vi "Process.vi"(8 "error in":errorcluster, 11 "Instrument.Example":refnum<class "Instrument.Oxford1820.lvclass">) -> (0 "error out":errorcluster, 3 "Instrument.Example out":refnum<class "Instrument.Oxford1820.lvclass">)   [LabVIEW 2016, in "Instrument.Oxford1820.lvclass"]
doc: "---------------------------------------------------------------\nJKI State Machine Objects™\nhttp://jki.net/state-machine-objects/\nCopyright (C) 2005-2015, JKI <info@jki.net>\nALL RIGHTS RESERVED"
uses:
  Instrument.Oxford1820.lvclass
  C:/Program Files (x86)/National Instruments/LabVIEW 2016/vi.lib/JKI/JKI SMO/SMO/SMO.lvclass
  <vilib>/JKI/JKI SMO/SMO/Typedefs/Parent Call--Enum.ctl
  <instrlib>/Mercury iXX/Public/Libraries/Magnet/Controls/Switch Heater.ctl
  <userlib>/LevyLab/Levylab Instruments/Instrument Types/Cryostat/Instrument.Cryostat.lvclass
  <vilib>/JKI/JKI SMO/SMO/SMO.lvclass
  <instrlib>/Mercury iXX/Public/Libraries/Magnet.lvlib
panel:
  # "For instructions on how to use the JKI State Machine Objects, examples and video tutorials, visit:\nhttp://jki.net/state-machine-objects/\n\nJKI State Machine Objects™\nhttp://jki.net/state-machine-objects/\nCopyright (C) 2005-2015, JKI <info@jki.net>\nALL RIGHTS RESERVED"
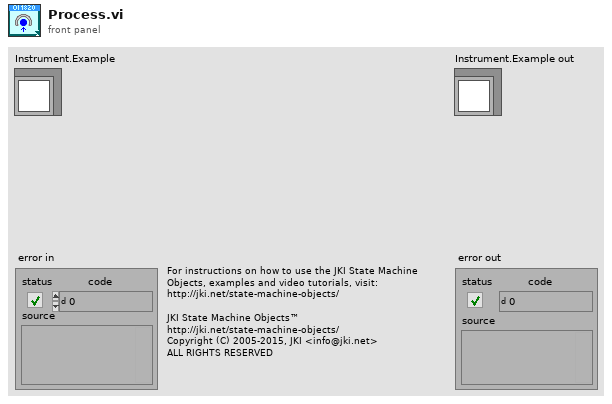
[diagram p1: front panel]
types:
  T1 = typedef "SMO.lvclass/Parent Call--Enum.ctl" = enum16{"Allows parent to run", "Does not request parent to run"}
  T2 = enum32{"invalid app kind", "Development System", "Run Time System", "Student Edition", "Embedded LabVIEW", "Evaluation", "Custom"}
  T3 = enum32{"Invalid", "Standard", "Closed", "Hidden", "Minimized", "Maximized"}
  T4 = enum32{"Bad", "Idle", "Run top level", "Running"}
  T5 = typedef "Mercury iXX.lvlib/Magnet.lvlib/Switch Heater.ctl" = string
  T6 = cluster{"Core":cluster{"Current VI Reference":refnum<vi>, "Close Panel on Exit?":bool, "error":errorcluster}, "Self Reference":refnum<class "Instrument.Oxford1820.lvclass">, "Field (T)":dbl, "Field Rate (T/min)":dbl, "persistent":bool, "Running Step":i32, "sequence":string[]}
  T7 = cluster{"Current VI Reference":refnum<vi>, "Close Panel on Exit?":bool, "error":errorcluster}
  T8 = typedef "SMO.lvclass/Protected Events.ctl" = cluster{"StopProcesses":refnum<user-event>, "AbortProcesses":refnum<user-event>, "Config Changed":refnum<user-event>, "Dependency":refnum<user-event>}
  T9 = typedef "Instrument.Oxford1820.lvclass/PrivateEvents--Cluster.ctl" = cluster{"SequenceSetMagnetField":refnum<user-event>}
  T10 = cluster{"Holding":bool, "Ramp to Setpoint":bool, "Ramp to Zero":bool, "Clamp":bool}
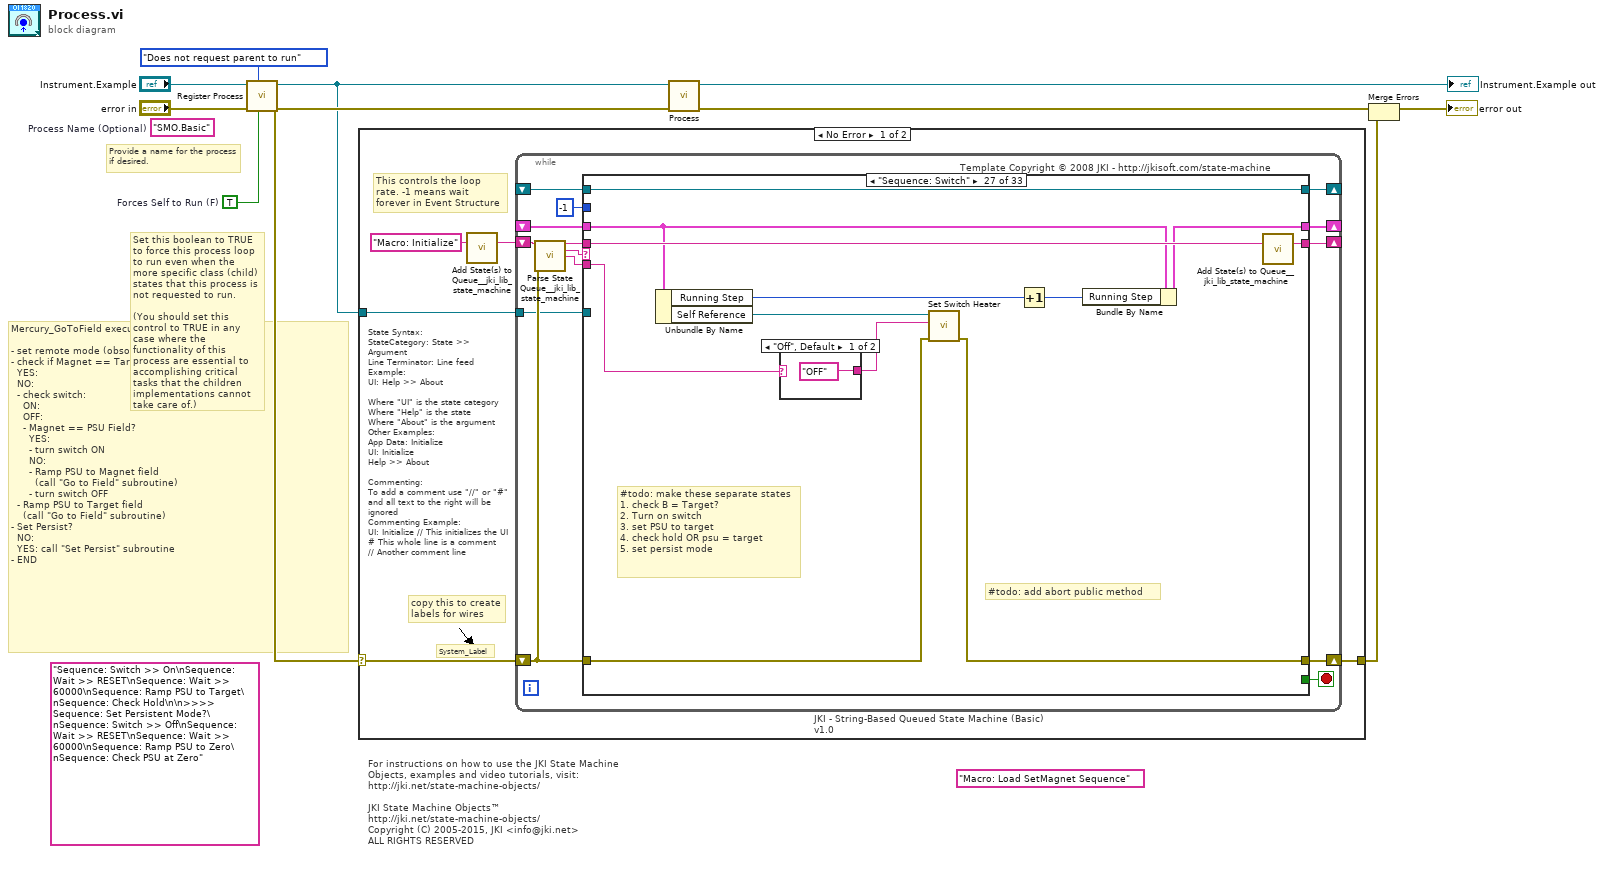
[diagram p0: block diagram]
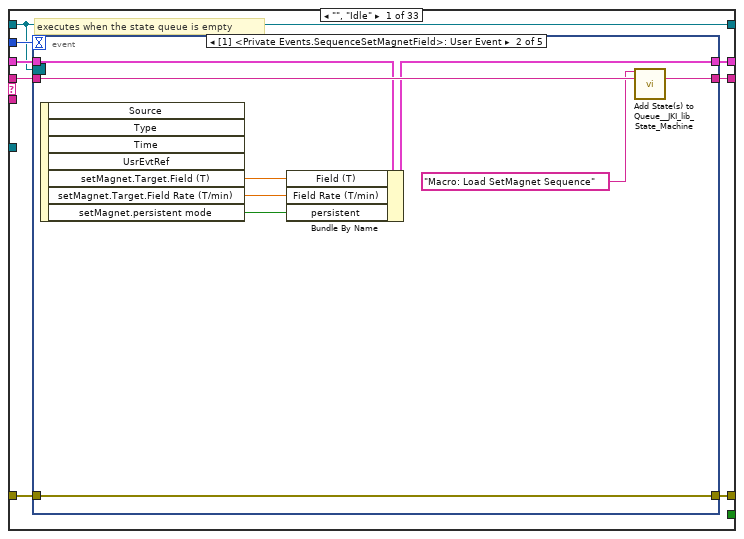
[diagram p2: hidden frame]
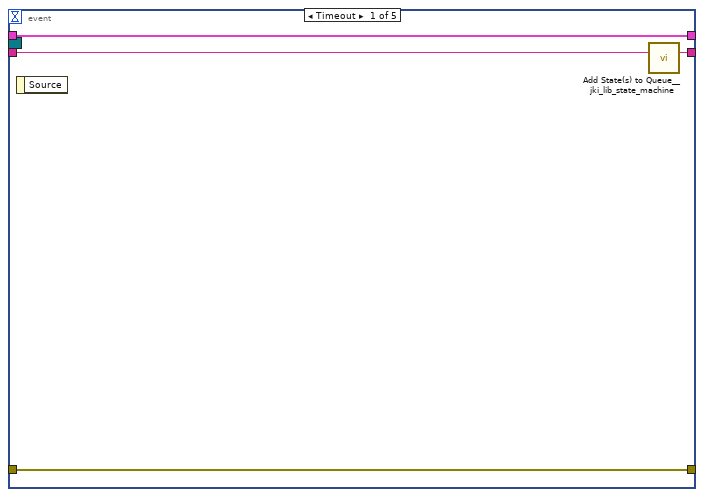
[diagram p3: hidden frame]
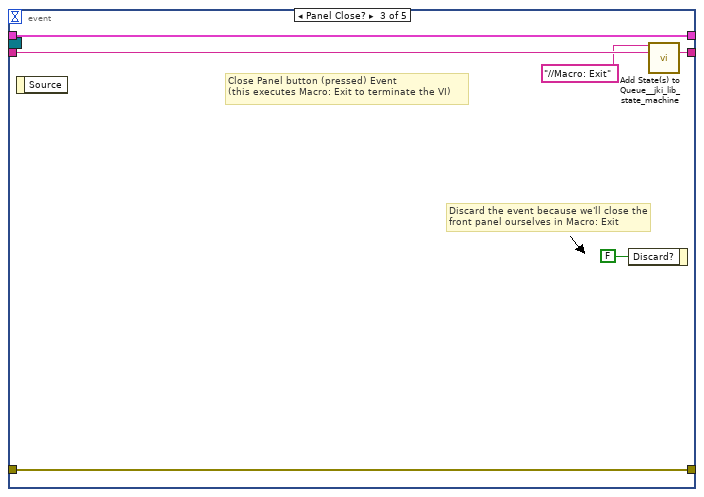
[diagram p4: hidden frame]
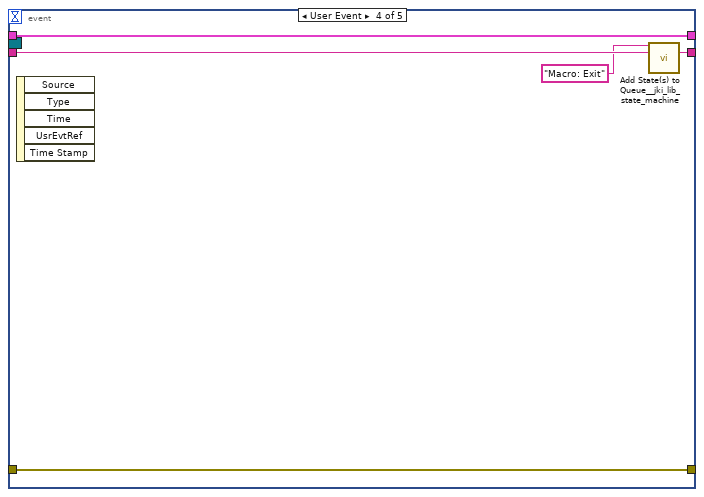
[diagram p5: hidden frame]
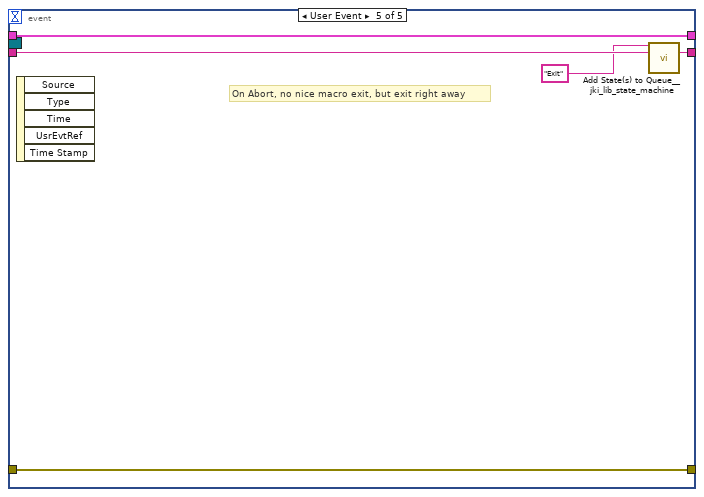
[diagram p6: hidden frame]
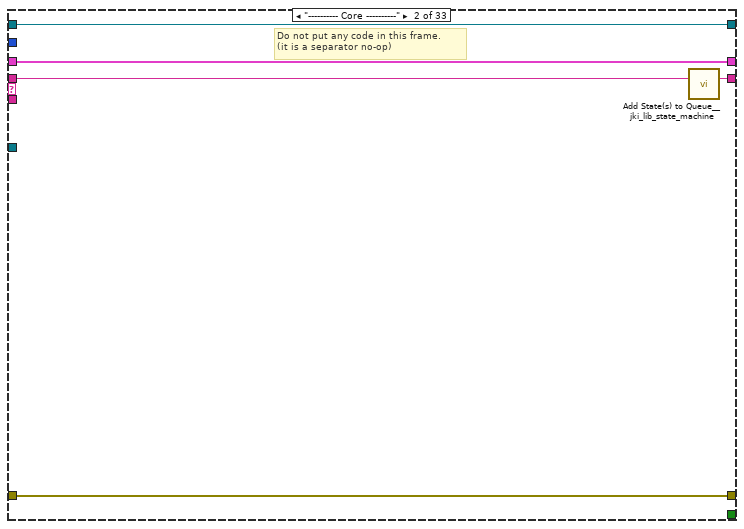
[diagram p7: hidden frame]
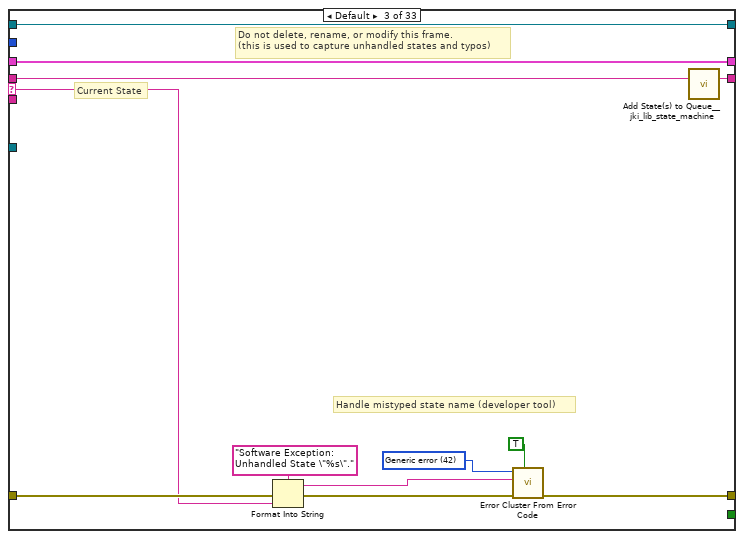
[diagram p8: hidden frame]
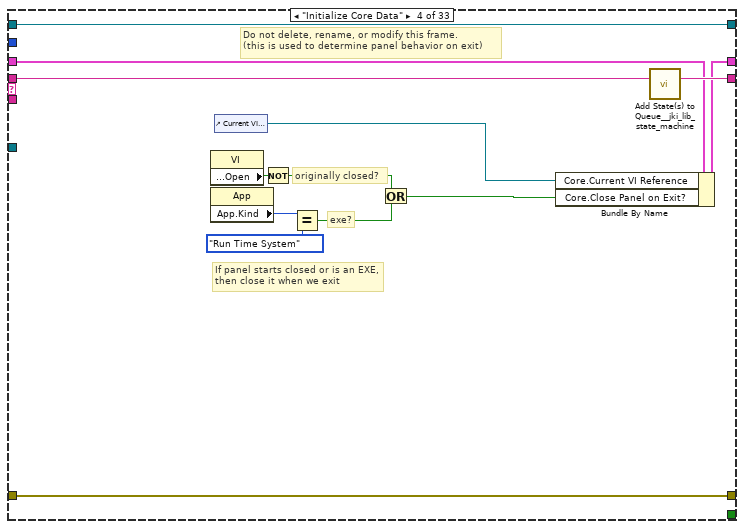
[diagram p9: hidden frame]
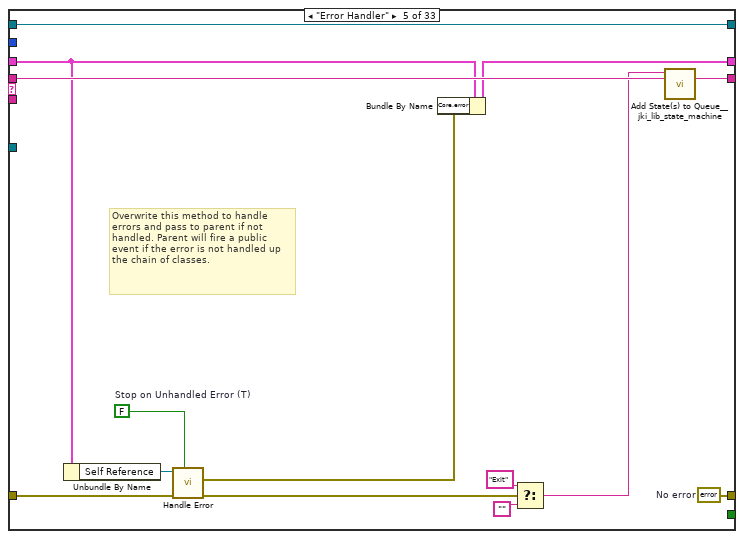
[diagram p10: hidden frame]
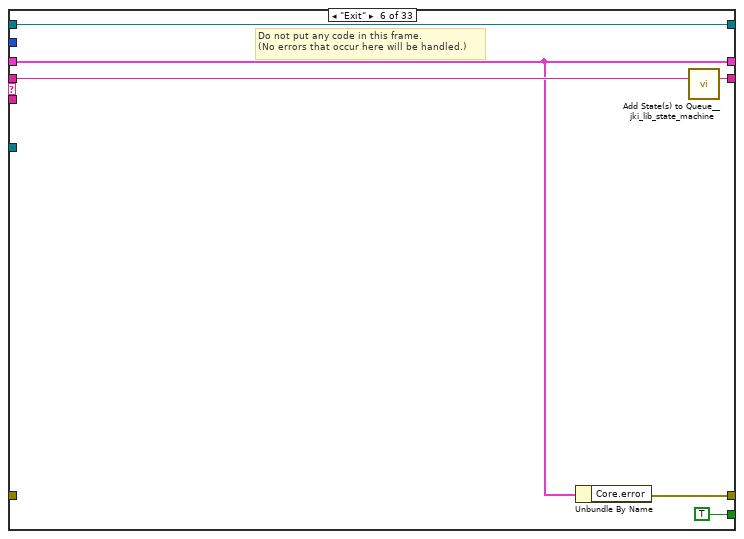
[diagram p11: hidden frame]
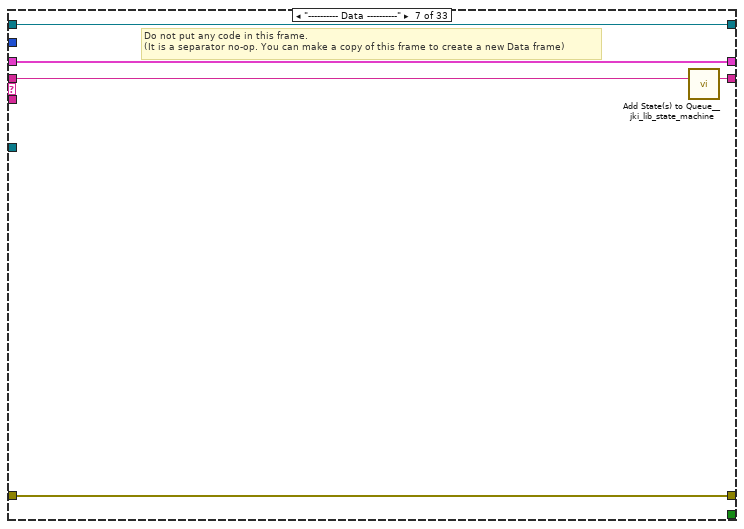
[diagram p12: hidden frame]
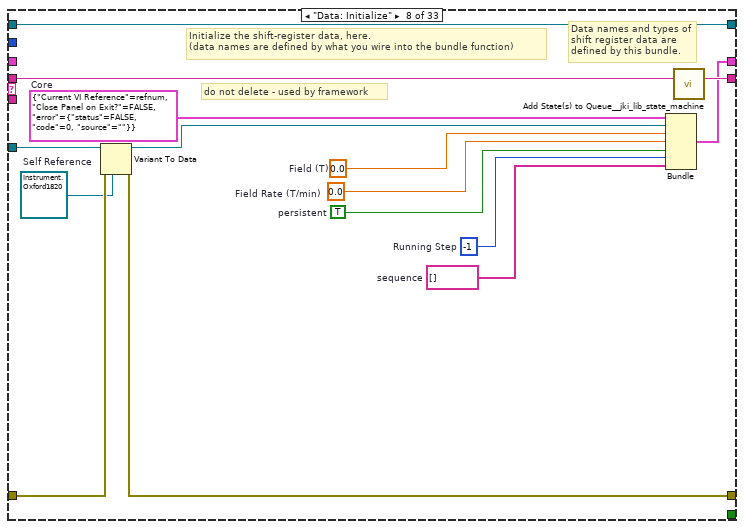
[diagram p13: hidden frame]
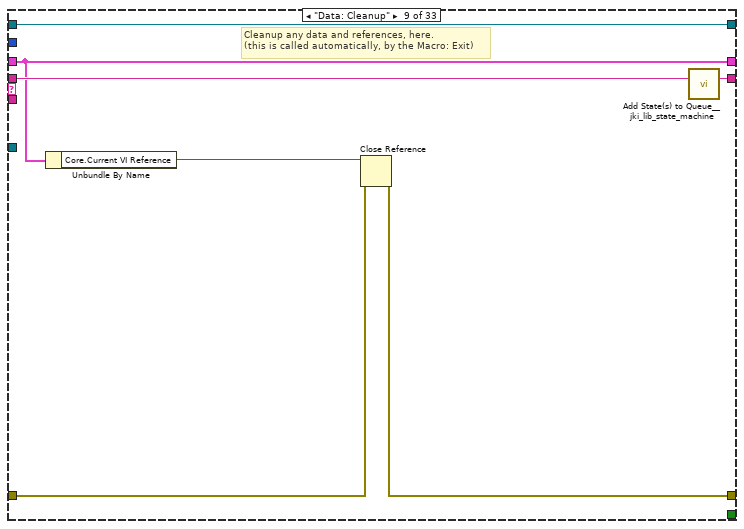
[diagram p14: hidden frame]
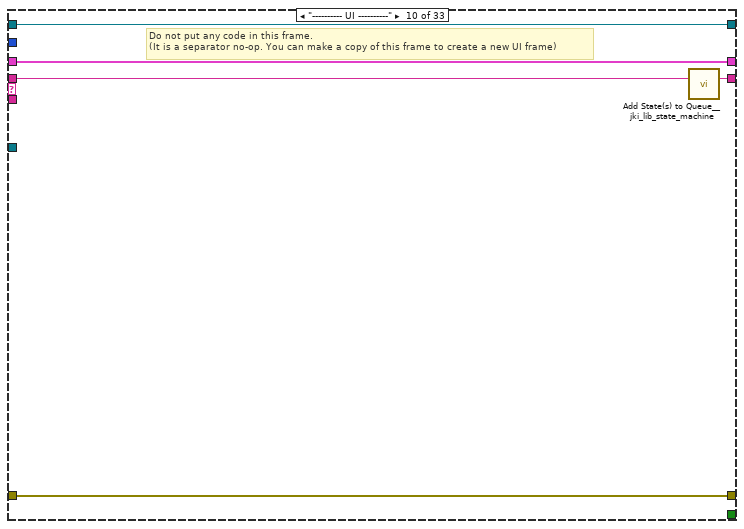
[diagram p15: hidden frame]
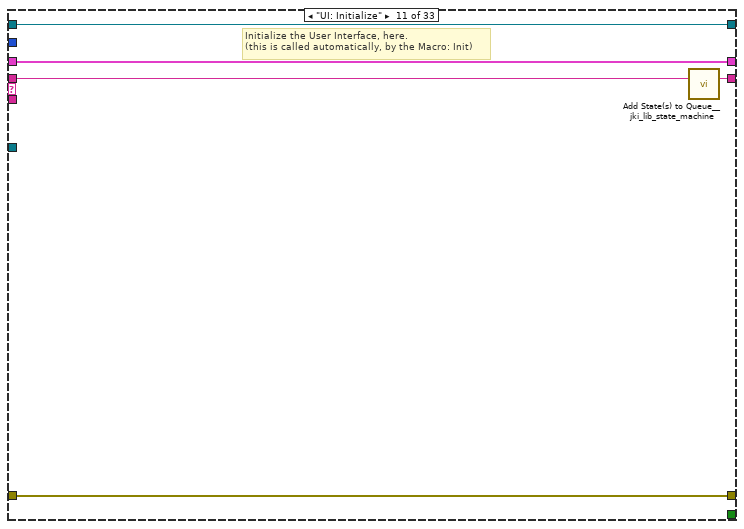
[diagram p16: hidden frame]
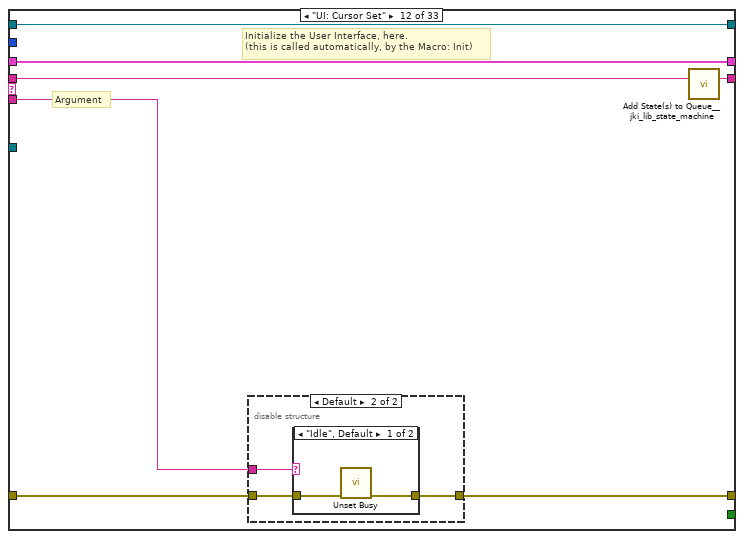
[diagram p17: hidden frame]
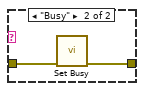
[diagram p19: hidden frame]
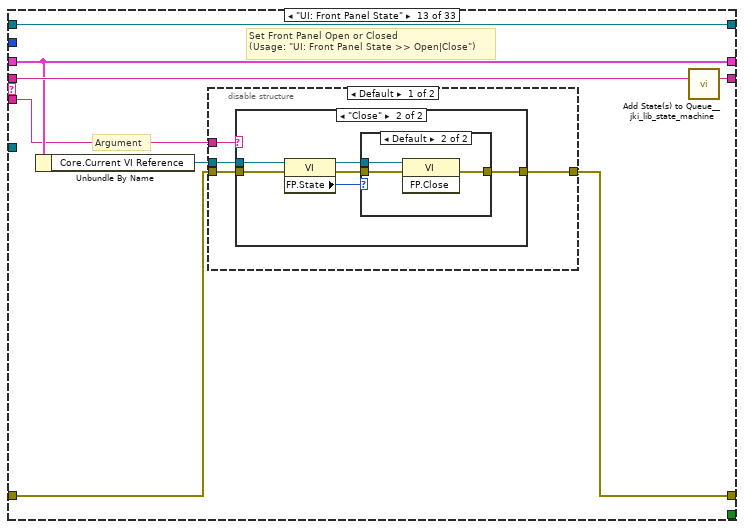
[diagram p20: hidden frame]
diagram:
  (unwired) "Macro: Load SetMagnet Sequence" ("State(s) at Back (\"\")")
  (unwired) "Sequence: Switch >> On\nSequence: Wait >> RESET\nSequence: Wait >> 60000\nSequence: Ramp PSU to Target\nSequence: Check Hold\n\n>>>> Sequence: Set Persistent Mode?\nSequence: Switch >> Off\nSequence: Wait >> RESET\nSequence: Wait >> 60000\nSequence: Ramp PSU to Zero\nSequence: Check PSU at Zero" ("State(s) in Front (\"\")")
  w1 = TRUE  # Forces Self to Run (F)
  (unwired) "SMO.Basic"  # Process Name (Optional)
  # "Mercury_GoToField executes the following states:\n\n- set remote mode (obsolete?)\n- check if Magnet == Target.\n  YES:\n  NO:\n  - check switch:\n    ON:\n    OFF:\n    - Magnet == PSU Field?\n      YES:\n      - turn switch ON\n      NO:\n      - Ramp PSU to Magnet field\n        (call \"Go to Field\" subroutine)\n      - turn switch OFF\n  - Ramp PSU to Target field\n    (call \"Go to Field\" subroutine)\n- Set Persist?\n  NO:\n  YES: call \"Set Persist\" subroutine\n- END"
  # "Provide a name for the process\nif desired."
  # "Set this boolean to TRUE to force this process loop to run even when the more specific class (child) states that this process is not requested to run.\n\n(You should set this control to TRUE in any case where the functionality of this process are essential to accomplishing critical tasks that the children implementations cannot take care of.)"
  # "For instructions on how to use the JKI State Machine Objects, examples and video tutorials, visit:\nhttp://jki.net/state-machine-objects/\n\nJKI State Machine Objects™\nhttp://jki.net/state-machine-objects/\nCopyright (C) 2005-2015, JKI <info@jki.net>\nALL RIGHTS RESERVED"
  n1 = call <vilib>:"Register Process.vi"("Forces Self to Run (F)"=w1, "Parent Call"=Parent_Call--Enum."Does not request parent to run", "error in (no error)"="error in", "SMO"="Instrument.Example") -> ("error out"=w7:errorcluster, "SMO out"=w6:refnum<class "Instrument.Oxford1820.lvclass">)  [unwired: 6 in]
  n2 = case shown="No Error" w7 {
    selector: w7 -> [w12 w472]
    tunnel: w6 -> [w13 _]
    tunnel: [w11 w472] -> w3
    frame No Error {
      # "State Syntax:\nStateCategory: State >> Argument\nLine Terminator: Line feed\nExample:\nUI: Help >> About\n\nWhere \"UI\" is the state category\nWhere \"Help\" is the state\nWhere \"About\" is the argument\nOther Examples:\nApp Data: Initialize\nUI: Initialize\nHelp >> About\n\nCommenting:\nTo add a comment use \"//\" or \"#\" and all text to the right will be ignored\nCommenting Example:\nUI: Initialize // This initializes the UI\n# This whole line is a comment\n// Another comment line"
      # "copy this to create labels for wires"
      # "This controls the loop rate. -1 means wait forever in Event Structure"
      # "System_Label"
      n3 = call <vilib>:"Add State(s) to Queue__jki_lib_state_machine.vi"("State(s) in (\"\")"="Macro: Initialize") -> ("States Out"=w15:string)  [unwired: 14 in]
      n4 = while "JKI - String-Based Queued State Machine (Basic) v1.0" {
        shift-right: [w22] -> _
        shift-left: _ -> [w21]
        shift-right: [w25] -> w11
        shift-left: w12 -> [w19]
        shift-right: [w24] -> _
        shift-left: w15 -> [w26]
        tunnel: w13 -> [w18]
        shift-right: [w17] -> _
        shift-left: _ -> [w16]
        stop <- w23 stop-if-true
        # "Template Copyright © 2008 JKI - http://jkisoft.com/state-machine"
        n5 = call <vilib>:"Parse State Queue__jki_lib_state_machine.vi"("State Queue"=w26, "Error In (no error)"=w19) -> ("Remaining States"=w28:string, "Current State"=w29:string, "Arguments"=w27:string)  [unwired: 11 in]
        n6 = case shown="\"Sequence: Switch\"" w29 {
          selector: w29 -> [_ _ w73 _ _ _ _ _ _ _ _ _ _ _ _ _ _ _ _ _ _ _ _ _ _ _ _ _ _ _ _ _ _]
          tunnel: w28 -> [w37 w71 w77 w96 w110 w116 w121 w136 w143 w148 w153 w160 w176 w208 w222 w236 w253 w268 w273 w284 w289 w302 w308 w317 w324 w338 w370 w388 w412 w432 w445 w459 w467]
          tunnel: w27 -> [_ _ _ _ _ _ _ _ _ _ _ w154 w170 _ _ _ _ _ _ _ _ _ _ _ _ _ w361 w373 _ _ _ _ _]
          tunnel: w21 -> [w35 w68 w75 w87 w104 w112 w118 _ w138 w145 w151 w158 w172 w205 w218 w227 w238 w264 w270 w281 w286 w300 w306 w311 w320 w335 w363 w385 w404 w429 w435 w456 w464]
          tunnel: [w34 w69 w79 w93 w105 w111 w119 w132 w139 w146 w150 w155 w173 w206 w220 w234 w251 w266 w271 w275 w287 w295 w304 w314 w321 w325 w359 w376 w400 w423 w440 w450 w461] -> w25
          tunnel: w19 -> [w33 w69 w78 w93 w106 _ w119 w133 w140 w146 w150 w156 w174 w206 w220 w234 w251 w266 w271 w276 w287 w296 w304 w314 w321 w326 w367 w375 w406 w424 w441 w451 w462]
          tunnel: [w36 w70 w76 w95 w109 w115 w120 w135 w142 w147 w152 w159 w175 w207 w221 w235 w252 w267 w272 w283 w288 w301 w307 w316 w323 w337 w369 w387 w411 w431 w444 w458 w466] -> w24
          tunnel: [_ _ _ _ _ TRUE _ _ _ _ _ _ _ _ _ _ _ _ _ _ _ _ _ _ _ _ _ _ _ _ _ _ _] -> w23
          tunnel: [w32 w68 w75 w94 w103 w112 w118 w134 w138 w145 w151 w158 w172 w205 w218 w227 w249 w262 w270 w281 w286 w300 w306 w310 w319 w335 w362 w384 w403 w428 w433 w455 w464] -> w22
          tunnel: -1 ("Timeout") -> [w31 _ _ _ _ _ _ _ _ _ _ _ _ _ _ _ _ _ _ _ _ _ _ _ _ _ _ _ _ _ _ _ _]
          tunnel: w18 -> [_ _ _ _ _ _ _ w130 _ _ _ _ _ _ _ _ _ _ _ _ _ _ _ _ _ _ _ _ _ _ _ _ _]
          tunnel: [w30 w67 w72 w84 w108 w113 w117 w128 w137 w144 w149 w157 w169 w204 w219 w228 w250 w265 w269 w282 w285 w299 w305 w315 w322 w336 w368 w386 w410 w430 w443 w457 w465] -> w17
          tunnel: w16 -> [w30 w67 w72 w84 w108 w113 w117 w128 w137 w144 w149 w157 w169 w204 w219 w228 w250 w265 w269 w282 w285 _ w305 w315 w322 w336 w368 w386 w410 w430 w443 w457 w465]
          frame "", "Idle" {
            # "executes when the state queue is empty"
            n7 = event shown="[1] <Private Events.SequenceSetMagnetField>: User Event" {
              selector: w30 -> [_ _ _ _ _]
              dyn-events: _ -> [_ _ _ _ _]
              timeout: w31 -> [_ _ _ _ _]
              tunnel: w37 -> [w41 w48 w56 w61 w66]
              tunnel: [w40 w49 w55 w60 w65] -> w36
              tunnel: w35 -> [w38 w44 w53 w58 w63]
              tunnel: [w39 w50 w54 w59 w64] -> w34
              tunnel: w33 -> [w39 w50 w54 w59 w64]
              tunnel: [w38 w43 w53 w58 w63] -> w32
              event Timeout {
                n8 = event-data() -> ()  [unwired: 1 in, 1 out]
                n9 = call <vilib>:"Add State(s) to Queue__jki_lib_state_machine.vi"("State(s) in (\"\")"=w41) -> ("States Out"=w40:string)  [unwired: 14 in]
              }
              event User Event {
                n10 = event-data() -> ("setMagnet.Target.Field (T)"=w47:dbl, "setMagnet.Target.Field Rate (T/min)"=w46:dbl, "setMagnet.persistent mode"=w45:bool)  [unwired: 1 in, 4 out]
                n11 = Bundle By Name(cluster=w44, "Field (T)"=w47, "Field Rate (T/min)"=w46, "persistent"=w45) -> (w43:T6)
                n12 = call <vilib>:"Add State(s) to Queue__JKI_lib_State_Machine.vi"("State(s) in Front (\"\")"="Macro: Load SetMagnet Sequence" ("State(s) at Back (\"\")"), "State(s) in (\"\")"=w48) -> ("States Out"=w49:string)  [unwired: 13 in]
              }
              event Panel Close? {
                # "Discard the event because we'll close the front panel ourselves in Macro: Exit"
                # "Close Panel button (pressed) Event\n(this executes Macro: Exit to terminate the VI)"
                n13 = event-data() -> ()  [unwired: 1 in, 1 out]
                n14 = event-data("Discard?"=FALSE) -> ()  [unwired: 1 in, 1 out]
                n15 = call <vilib>:"Add State(s) to Queue__jki_lib_state_machine.vi"("State(s) in Front (\"\")"="//Macro: Exit", "State(s) in (\"\")"=w56) -> ("States Out"=w55:string)  [unwired: 13 in]
              }
              event User Event {
                n16 = event-data() -> ()  [unwired: 1 in, 5 out]
                n17 = call <vilib>:"Add State(s) to Queue__jki_lib_state_machine.vi"("State(s) in Front (\"\")"="Macro: Exit", "State(s) in (\"\")"=w61) -> ("States Out"=w60:string)  [unwired: 13 in]
              }
              event User Event {
                # "On Abort, no nice macro exit, but exit right away"
                n18 = event-data() -> ()  [unwired: 1 in, 5 out]
                n19 = call <vilib>:"Add State(s) to Queue__jki_lib_state_machine.vi"("State(s) in Front (\"\")"="Exit", "State(s) in (\"\")"=w66) -> ("States Out"=w65:string)  [unwired: 13 in]
              }
            }
          }
          frame "---------- Core ----------" {
            # "Do not put any code in this frame.\n(it is a separator no-op)"
            n20 = call <vilib>:"Add State(s) to Queue__jki_lib_state_machine.vi"("State(s) in (\"\")"=w71) -> ("States Out"=w70:string)  [unwired: 14 in]
          }
          frame Default {
            w82 = 42 items=["No error", "Argument error", "Memory is full", "Out of zone", "End of file", "File already open", "Generic file I/O error", "File not found", "File permission error", "Disk is full", "Duplicate path", "Too many files open", "System feature not enabled", "Resource file not found", "Cannot add resource", "Resource not found", "Image not found", "Image memory error", "Pen does not exist", "Config type invalid", "Config token not found", "Config parse error", "Config memory error", "Bad external code format", "Bad external code offset", "External code not present", "Null window", "Destroy window error", "Null menu", "Print aborted", "Bad print record", "Print driver error", "Windows error during printing", "Memory error during printing", "Print dialog error", "Generic print error", "Invalid device refnum", "Device not found", "Device parameter error", "Device unit error", "Cannot open device", "Device call aborted", "Generic error", "Cancelled by user", "Object ID too low", "Object ID too high", "Object not in heap", "Unknown heap", "Unknown object (invalid DefProc)", "Unknown object (DefProc not in table)", "Message out of range", "Invalid (null) method", "Unknown message", "Manager call not supported", "Bad address", "Network operation in progress", "Network operation timed out", "Connection is busy", "Network attribute not supported", "Network error", "Address in use", "System out of memory", "Connection aborted", "Connection refused", "Not connected", "Already connected", "Connection closed", "Initialization error (interapplication manager)", "Bad occurrence", "Wait on unbound occurrence handler", "Occurrence queue overflow", "Datalog type conflict", "Unused", "Unrecognized type (interapplication manager)", "Memory corrupt", "Failed to make temporary DLL", "Old CIN version", "Drag socket not found", "Failed to load drop-object", "Failed to register OLE object", "Failed to release OLE object", "Format specifier type mismatch", "Unknown format specifier", "Too few format specifiers", "Too many format specifiers", "Scan failed", "Newer CIN version", "Error converting to variant", "Runtime menu error", "Password tampered", "Variant attribute not found", "Incompatible variant data type", "Event data is not available", "Event Store is not present", "Occurrence is not found", "Event Queue is not created", "Event info is not available", "Refnum passed is NULL", "Error retrieving Class GUID", "Error retrieving CoClass GUID", "Error retrieving TypeLib GUID.", "Bad built application magic bytes.", "Specific driver is different from the specific driver associated with the Logical Name.", "There is no session opened to the class driver.", "Max Error", "MAX - Error with config objects", "MAX - Error loading configuration", "MAX - Group not supported"]
            # "Current State"
            # "Do not delete, rename, or modify this frame.\n(this is used to capture unhandled states and typos)"
            # "Handle mistyped state name (developer tool)"
            n21 = Format Into String(format string="Software Exception: Unhandled State \"%s\"." ("message"), error in=w78, w73) -> (resulting string=w81:string, error out=w80:errorcluster)  [unwired: 1 in]
            n22 = call <vilib>:"Error Cluster From Error Code.vi"("show call chain? (False)"=TRUE, "error in (no error)"=w80, "error message (\"\")"=w81, "error code (0)"=w82) -> ("error out"=w79:errorcluster)  [unwired: 5 in]
            n23 = call <vilib>:"Add State(s) to Queue__jki_lib_state_machine.vi"("State(s) in (\"\")"=w77) -> ("States Out"=w76:string)  [unwired: 14 in]
          }
          frame "Initialize Core Data" {
            # "Do not delete, rename, or modify this frame.\n(this is used to determine panel behavior on exit)"
            # "originally closed?"
            # "exe?"
            # "If panel starts closed or is an EXE, then close it when we exit"
            n24 = property class="VI"() -> ("Front Panel.Open"=w92:bool)  [unwired: 2 in, 2 out]
            n25 = property class="App"() -> ("App.Kind"=w91:T2)  [unwired: 2 in, 2 out]
            n26 = control-ref of="Current VI Reference"() -> (w85:refnum<vi>)
            n27 = Not(x=w92) -> (.not. x?=w89:bool)
            n28 = Equal?(x=w91, y=T2."Run Time System" ("Application:Kind")) -> (x = y?=w88:bool)
            n29 = Or(x=w89, y=w88) -> (x .or. y?=w86:bool)
            n30 = Bundle By Name(cluster=w87, "Core.Current VI Reference"=w85, "Core.Close Panel on Exit?"=w86) -> (w94:T6)
            n31 = call <vilib>:"Add State(s) to Queue__jki_lib_state_machine.vi"("State(s) in (\"\")"=w96) -> ("States Out"=w95:string)  [unwired: 14 in]
          }
          frame "Error Handler" {
            w97 = FALSE  # Stop on Unhandled Error (T)
            w105 = errorcluster {"status"=FALSE, "code"=0, "source"=""}  # No error
            # "Overwrite this method to handle errors and pass to parent if not handled. Parent will fire a public event if the error is not handled up the chain of classes."
            n32 = Unbundle By Name(w104) -> ("Self Reference"=w107:refnum<class "Instrument.Oxford1820.lvclass">)
            n33 = call-dynamic "Handle Error.vi"("Stop on Unhandled Error (T)"=w97, "error in"=w106, "LevyLab"=w107) -> ("handling error"=w98:errorcluster, "Unhandled error"=w101:errorcluster)  [unwired: 6 in, 1 out]
            n34 = Bundle By Name(cluster=w104, "Core.error"=w101) -> (w103:T6)
            n35 = Select(t="Exit", s=w98, f="") -> (s? t:f=w102:string)
            n36 = call <vilib>:"Add State(s) to Queue__jki_lib_state_machine.vi"("State(s) in Front (\"\")"=w102, "State(s) in (\"\")"=w110) -> ("States Out"=w109:string)  [unwired: 13 in]
          }
          frame "Exit" {
            # "Do not put any code in this frame.\n(No errors that occur here will be handled.)"
            n37 = Unbundle By Name(w112) -> ("Core.error"=w111:errorcluster)
            n38 = call <vilib>:"Add State(s) to Queue__jki_lib_state_machine.vi"("State(s) in (\"\")"=w116) -> ("States Out"=w115:string)  [unwired: 14 in]
          }
          frame "---------- Data ----------" {
            # "Do not put any code in this frame.\n(It is a separator no-op. You can make a copy of this frame to create a new Data frame)"
            n39 = call <vilib>:"Add State(s) to Queue__jki_lib_state_machine.vi"("State(s) in (\"\")"=w121) -> ("States Out"=w120:string)  [unwired: 14 in]
          }
          frame "Data: Initialize" {
            w122 = string[] []  # sequence
            w123 = -1  # Running Step
            w124 = TRUE  # persistent
            w125 = 0.0  # Field Rate (T/min)
            w126 = 0.0  # Field (T)
            w127 = T7 {"Current VI Reference"=refnum, "Close Panel on Exit?"=FALSE, "error"={"status"=FALSE, "code"=0, "source"=""}}  # Core
            w131 = refnum<class "Instrument.Oxford1820.lvclass"> refnum  # Self Reference
            # "do not delete - used by framework"
            # "Data names and types of shift register data are defined by this bundle."
            # "Initialize the shift-register data, here.\n(data names are defined by what you wire into the bundle function)"
            n40 = Variant To Data(error in=w133, type=w131, Variant=w130) -> (data=w129:refnum<class "Instrument.Oxford1820.lvclass">, error out=w132:errorcluster)
            n41 = Bundle("Core"=w127, "Self Reference"=w129, "Field (T)"=w126, "Field Rate (T/min)"=w125, "persistent"=w124, "Running Step"=w123, "sequence"=w122) -> (w134:T6)  [unwired: 1 in]
            n42 = call <vilib>:"Add State(s) to Queue__jki_lib_state_machine.vi"("State(s) in (\"\")"=w136) -> ("States Out"=w135:string)  [unwired: 14 in]
          }
          frame "Data: Cleanup" {
            # "Cleanup any data and references, here.\n(this is called automatically, by the Macro: Exit)"
            n43 = Unbundle By Name(w138) -> ("Core.Current VI Reference"=w141:refnum<vi>)
            n44 = Close Reference(reference=w141, error in (no error)=w140) -> (error out=w139:errorcluster)
            n45 = call <vilib>:"Add State(s) to Queue__jki_lib_state_machine.vi"("State(s) in (\"\")"=w143) -> ("States Out"=w142:string)  [unwired: 14 in]
          }
          frame "---------- UI ----------" {
            # "Do not put any code in this frame.\n(It is a separator no-op. You can make a copy of this frame to create a new UI frame)"
            n46 = call <vilib>:"Add State(s) to Queue__jki_lib_state_machine.vi"("State(s) in (\"\")"=w148) -> ("States Out"=w147:string)  [unwired: 14 in]
          }
          frame "UI: Initialize" {
            # "Initialize the User Interface, here.\n(this is called automatically, by the Macro: Init)"
            n47 = call <vilib>:"Add State(s) to Queue__jki_lib_state_machine.vi"("State(s) in (\"\")"=w153) -> ("States Out"=w152:string)  [unwired: 14 in]
          }
          frame "UI: Cursor Set" {
            # "Argument"
            # "Initialize the User Interface, here.\n(this is called automatically, by the Macro: Init)"
            n48 = disable-structure shown="Default" {
              disable-tunnel: w156 -> [w161 w164]
              disable-tunnel: [w161 w163] -> w155
              disable-tunnel: w154 -> [_ w162]
              frame condition #0 {
              }
              frame condition #1 (active) {
                n49 = case shown="\"Idle\", Default" w162 {
                  tunnel: w164 -> [w166 w168]
                  tunnel: [w165 w167] -> w163
                  frame "Idle", Default {
                    n50 = call <vilib>:"Unset Busy.vi"("error in (no error)"=w166) -> ("error out"=w165:errorcluster)  [unwired: 10 in]
                  }
                  frame "Busy" {
                    n51 = call <vilib>:"Set Busy.vi"("error in (no error)"=w168) -> ("error out"=w167:errorcluster)  [unwired: 9 in, 1 out]
                  }
                }
              }
            }
            n52 = call <vilib>:"Add State(s) to Queue__jki_lib_state_machine.vi"("State(s) in (\"\")"=w160) -> ("States Out"=w159:string)  [unwired: 14 in]
          }
          frame "UI: Front Panel State" {
            # "Argument"
            # "Set Front Panel Open or Closed\n(Usage: \"UI: Front Panel State >> Open|Close\")"
            n53 = Unbundle By Name(w172) -> ("Core.Current VI Reference"=w171:refnum<vi>)
            n54 = disable-structure shown="Default" {
              disable-tunnel: w174 -> [w180 w203]
              disable-tunnel: [w179 w203] -> w173
              disable-tunnel: w171 -> [w178 _]
              disable-tunnel: w170 -> [w177 _]
              frame condition #0 (active) {
                n55 = case shown="\"Close\"" w177 {
                  tunnel: w180 -> [w184 w197]
                  tunnel: [w186 w198] -> w179
                  tunnel: w178 -> [w185 w195]
                  frame "Open", Default {
                    n56 = property class="VI"(reference=w185, error in=w184) -> (reference out=w182:refnum<vi>, error out=w183:errorcluster, "FP.State"=w181:T3)
                    n57 = case shown="\"Closed\"" w181 {
                      tunnel: [w189 w192] -> w186
                      tunnel: w183 -> [w188 w192]
                      tunnel: w182 -> [w187 _]
                      frame "Closed" {
                        n58 = invoke class="VI" method="FP.Open"(reference=w187, error in=w188, "Activate"=TRUE, "State"=T3."Standard") -> (error out=w189:errorcluster)  [unwired: 1 in, 4 out]
                      }
                      frame Default {
                      }
                    }
                  }
                  frame "Close" {
                    n59 = property class="VI"(reference=w195, error in=w197) -> (reference out=w194:refnum<vi>, error out=w196:errorcluster, "FP.State"=w193:T3)
                    n60 = case shown="Default" w193 {
                      tunnel: [w199 w202] -> w198
                      tunnel: w196 -> [w199 w201]
                      tunnel: w194 -> [_ w200]
                      frame "Invalid", "Closed" {
                      }
                      frame Default {
                        n61 = invoke class="VI" method="FP.Close"(reference=w200, error in=w201) -> (error out=w202:errorcluster)  [unwired: 1 in, 2 out]
                      }
                    }
                  }
                }
              }
              frame condition #1 {
              }
            }
            n62 = call <vilib>:"Add State(s) to Queue__jki_lib_state_machine.vi"("State(s) in (\"\")"=w176) -> ("States Out"=w175:string)  [unwired: 14 in]
          }
          frame "---------- Macro ----------" {
            # "Do not put any code in this frame.\n(It is a separator no-op. You can make a copy of this frame to create a new Macro frame)"
            n63 = call <vilib>:"Add State(s) to Queue__jki_lib_state_machine.vi"("State(s) in (\"\")"=w208) -> ("States Out"=w207:string)  [unwired: 14 in]
          }
          frame "Macro: Initialize" {
            w213 = "//UI: Initialize\n//UI: Front Panel State >> Open"  # //UI: Initialize //UI: Front Panel State >> Open
            w209 = "Process: Sync"
            # "Initialization Macro\n(This is called once, when the VI starts)"
            n64 = control-ref of="This VI"() -> (w211:refnum<vi>)
            n65 = property class="VI"(reference=w211) -> ("Exec.State"=w210:T4)  [unwired: 1 in, 2 out]
            n66 = Equal?(x=w210, y=T4."Run top level") -> (x = y?=w216:bool)
            n67 = Select(t=w209, s=w216, f="") -> ()  [unwired: 1 out]
            n68 = call <vilib>:"Add State(s) to Queue__jki_lib_state_machine.vi"("State(s) in Front (\"\")"="Data: Initialize\nInitialize Core Data\nEvents: Register", "State(s) in (\"\")"=w209, "State(s) at Back (\"\")"=w213) -> ("States Out"=w212:string)  [unwired: 12 in]
            n69 = call <vilib>:"Add State(s) to Queue__jki_lib_state_machine.vi"("State(s) in Front (\"\")"=w212, "State(s) in (\"\")"=w222) -> ("States Out"=w221:string)  [unwired: 13 in]
          }
          frame "Macro: Exit" {
            # "Exit Macro\n(This is called once, when the VI exits)"
            n70 = Unbundle By Name(w227) -> ("Core.Close Panel on Exit?"=w233:bool)
            n71 = Select(t="UI: Front Panel State >> Close", s=w233, f="") -> (s? t:f=w230:string)
            n72 = call <vilib>:"Add State(s) to Queue__jki_lib_state_machine.vi"("State(s) in Front (\"\")"="Data: Cleanup\nEvents: Unregister", "State(s) in (\"\")"="Process: Sync", "State(s) at Back (\"\")"="Exit") -> ("States Out"=w224:string)  [unwired: 12 in]
            n73 = call <vilib>:"Add State(s) to Queue__jki_lib_state_machine.vi"("State(s) in (\"\")"=w230, "State(s) at Back (\"\")"=w224) -> ("States Out"=w229:string)  [unwired: 13 in]
            n74 = call <vilib>:"Add State(s) to Queue__jki_lib_state_machine.vi"("State(s) in Front (\"\")"=w229, "State(s) in (\"\")"=w236) -> ("States Out"=w235:string)  [unwired: 13 in]
          }
          frame "Macro: Run Sequence" {
            # "0,1,2,3,4,"
            # "5"
            # "Do not put any code in this frame.\n(It is a separator no-op. You can make a copy of this frame to create a new Macro frame)"
            n75 = Unbundle By Name(w238) -> ("sequence"=w247:string[], "Running Step"=w237:i32)
            n76 = Array Size(array=w247) -> (size(s)=w248:i32)
            n77 = Index Array(array=w247, index=w237) -> (element=w244:string)
            n78 = Equal?(x=w248, y=w237) -> (x = y?=w241:bool)
            n79 = Select(t=-1 ("Running Step"), s=w241, f=w237) -> (s? t:f=w245:i32)
            n80 = Select(t="", s=w241, f="Macro: Run Sequence" ("State(s) at Back (\"\")")) -> (s? t:f=w239:string)
            n81 = Bundle By Name(cluster=w238, "Running Step"=w245) -> (w249:T6)
            n82 = call <vilib>:"Add State(s) to Queue__jki_lib_state_machine.vi"("State(s) in Front (\"\")"=w244, "State(s) at Back (\"\")"=w239) -> ("States Out"=w243:string)  [unwired: 13 in]
            n83 = call <vilib>:"Add State(s) to Queue__jki_lib_state_machine.vi"("State(s) in Front (\"\")"=w243, "State(s) in (\"\")"=w253) -> ("States Out"=w252:string)  [unwired: 13 in]
          }
          frame "Macro: Load SetMagnet Sequence" {
            # "Do not put any code in this frame.\n(It is a separator no-op. You can make a copy of this frame to create a new Macro frame)"
            n84 = Unbundle By Name(w264) -> ("persistent"=w261:bool)
            n85 = Select(t="Sequence: Switch >> Off\nSequence: Wait >> RESET\nSequence: Wait >> 60000\nSequence: Ramp PSU to Zero\nSequence: Check PSU at Zero" ("State(s) in Front (\"\")"), s=w261, f="") -> (s? t:f=w259:string)
            n86 = call <vilib>:"Add State(s) to Queue__jki_lib_state_machine.vi"("State(s) in Front (\"\")"="Sequence: Switch >> On\nSequence: Wait >> RESET\nSequence: Wait >> 60000\nSequence: Ramp PSU to Target\nSequence: Check Hold" ("State(s) in Front (\"\")"), "State(s) at Back (\"\")"=w259) -> ("States Out"=w257:string)  [unwired: 13 in]
            n87 = call <userlib>:"String to 1D Array__ogtk.vi"("string"=w257) -> ("Array of Strings"=w256:string[])  [unwired: 10 in]
            n88 = Bundle By Name(cluster=w264, "Running Step"=0 ("sequence"), "sequence"=w256) -> (w262:T6)
            n89 = call <vilib>:"Add State(s) to Queue__jki_lib_state_machine.vi"("State(s) in Front (\"\")"="Macro: Run Sequence" ("State(s) in Front (\"\")"), "State(s) in (\"\")"=w268) -> ("States Out"=w267:string)  [unwired: 13 in]
          }
          frame "---------- Process ----------" {
            # "Template Separator\n(You can make a copy of, or modify, this frame)"
            n90 = call <vilib>:"Add State(s) to Queue__jki_lib_state_machine.vi"("State(s) in (\"\")"=w273) -> ("States Out"=w272:string)  [unwired: 14 in]
          }
          frame "Process: Sync" {
            n91 = Unbundle By Name(w281) -> ("Self Reference"=w277:refnum<class "Instrument.Oxford1820.lvclass">)
            n92 = call <vilib>:"WaitOnProcessSync.vi"("error in (no error)"=w276, "SMO"=w277) -> ("error out"=w275:errorcluster, "Don't run?"=w280:bool)  [unwired: 7 in, 1 out]
            n93 = Select(t="Data: Cleanup\nEvents: Unregister\nExit", s=w280, f="") -> (s? t:f=w274:string)
            n94 = call <vilib>:"Add State(s) to Queue__jki_lib_state_machine.vi"("State(s) in Front (\"\")"=w274, "State(s) in (\"\")"=w284) -> ("States Out"=w283:string)  [unwired: 13 in]
          }
          frame "---------- Events ----------" {
            # "Template Separator\n(You can make a copy of, or modify, this frame)"
            n95 = call <vilib>:"Add State(s) to Queue__jki_lib_state_machine.vi"("State(s) in (\"\")"=w289) -> ("States Out"=w288:string)  [unwired: 14 in]
          }
          frame "Events: Register" {
            # "Expand to add\nmore events"
            n96 = Unbundle By Name(w300) -> ("Self Reference"=w297:refnum<class "Instrument.Oxford1820.lvclass">)
            n97 = call <vilib>:"GetProtectedEvents.vi"("SMO"=w297) -> ("error out"=w293:errorcluster, "SMO Protected Events"=w298:T8, "SMO out"=w292:refnum<class "Instrument.Oxford1820.lvclass">)  [unwired: 8 in]
            n98 = call "Instrument.Oxford1820.GetPrivateEvents.vi"("Instrument.Oxford1820"=w292) -> ("error out"=w290:errorcluster, "Private Events"=w291:T9)  [unwired: 8 in, 1 out]
            n99 = register-events(w298, w291) -> (reference out=w299:refnum<event-registration>, error out=w294:errorcluster)  [unwired: 2 in]
            n100 = Merge Errors(w290, w296, w294, w293) -> (w295:errorcluster)
            n101 = call <vilib>:"Add State(s) to Queue__jki_lib_state_machine.vi"("State(s) in (\"\")"=w302) -> ("States Out"=w301:string)  [unwired: 14 in]
          }
          frame "Events: Unregister" {
            n102 = Unregister For Events(event registration refnum=w305, error in=w304) -> (error out=w303:errorcluster)
            n103 = call <vilib>:"Clear Errors.vi"("error in (no error)"=w303) -> ()  [unwired: 5 in, 2 out]
            n104 = call <vilib>:"Add State(s) to Queue__jki_lib_state_machine.vi"("State(s) in (\"\")"=w308) -> ("States Out"=w307:string)  [unwired: 14 in]
          }
          frame "---------- Sequence ----------" {
            n105 = Unbundle By Name(w311) -> ("Running Step"=w309:i32, "Self Reference"=w313:refnum<class "Instrument.Oxford1820.lvclass">)
            n106 = Increment(x=w309) -> (x+1=w312:i32)
            n107 = Bundle By Name(cluster=w311, "Running Step"=w312, "Self Reference"=w313) -> (w310:T6)
            n108 = call <vilib>:"Add State(s) to Queue__jki_lib_state_machine.vi"("State(s) in (\"\")"=w317) -> ("States Out"=w316:string)  [unwired: 14 in]
          }
          frame "Sequence: Template" {
            # "switch ON/OFF:\n- include checks for PSU == Magnet.\n- call \"Go to Field\" as needed to make PSU == Magnet"
            # "\"Set Persist\" subroutine:\n\n- switch on?\n  NO:\n  YES:\n  - turn switch OFF\n- Ramp PSU to 0\n  (call \"Go to Field\" subroutine)\n- END"
            # "\"Go to Field\" subroutine:\n\n- set to remote mode (obsolete?)\n- write target field.\n  check and resend if necessary\n- put in hold mode.\n  check and resend if necessary\n- check if Target = PSU:\n  YES:\n  NO:\n  - put in GTOS mode. check and resend if necessary\n- wait until PSU is in hold mode\n  (PSU will go to hold mode once PSU @ target)\n- END"
            # "Mercury_GoToField executes the following states:\n\n- set remote mode (obsolete?)\n- check if Magnet == Target.\n  YES:\n  NO:\n  - check switch:\n    ON:\n    OFF:\n    - Magnet == PSU Field?\n      YES:\n      - turn switch ON\n      NO:\n      - Ramp PSU to Magnet field\n        (call \"Go to Field\" subroutine)\n      - turn switch OFF\n  - Ramp PSU to Target field\n    (call \"Go to Field\" subroutine)\n- Set Persist?\n  NO:\n  YES: call \"Set Persist\" subroutine\n- END"
            n109 = Unbundle By Name(w320) -> ("Self Reference"=w318:refnum<class "Instrument.Oxford1820.lvclass">)
            n110 = Bundle By Name(cluster=w320, "Self Reference"=w318) -> (w319:T6)
            n111 = call <vilib>:"Add State(s) to Queue__jki_lib_state_machine.vi"("State(s) in (\"\")"=w324) -> ("States Out"=w323:string)  [unwired: 14 in]
          }
          frame "Sequence: Sequence" {
            # "DELETE THIS STATE"
            # "#todo: add abort public method"
            # "#todo: make these separate states\n1. check B = Target?\n2. Turn on switch\n3. set PSU to target\n4. check hold OR psu = target\n5. set persist mode"
            n112 = Unbundle By Name(w335) -> ("Self Reference"=w334:refnum<class "Instrument.Oxford1820.lvclass">, "Field (T)"=w328:dbl, "Field Rate (T/min)"=w329:dbl, "persistent"=w327:bool)
            n113 = call-dynamic "Get Magnet Field.vi"("error in (no error)"=w326, "Instrument.Oxford1820 in"=w334) -> ("error out"=w331:errorcluster, "B Field (T)"=w333:dbl, "Instrument.Oxford1820 out"=w330:refnum<class "Instrument.Oxford1820.lvclass">)  [unwired: 5 in, 2 out]
            n114 = call "Instrument.1820.FloatApprox.vi"("y"=w328, "x"=w333) -> ("x ~ y?"=w332:bool)  [unwired: 4 in]
            n115 = case shown="False" w332 {
              tunnel: w331 -> [w349 w357]
              tunnel: w330 -> [w350 w358]
              tunnel: w329 -> [w344 _]
              tunnel: w328 -> [w345 _]
              tunnel: w327 -> [w343 _]
              tunnel: [w340 w357] -> w325
              tunnel: [w339 w358] -> _
              frame False {
                n116 = call "Set Switch Heater.vi"("error in (no error)"=w349, "Switch Heater"=T5 "ON", "Instrument.1820 in"=w350) -> ("error out"=w347:errorcluster, "Instrument.1820 in"=w346:refnum<class "Instrument.Oxford1820.lvclass">)  [unwired: 6 in, 1 out]
                n117 = call "Ramp PSU to Target.vi"("error in (no error)"=w347, "Target Rate (T/min)"=w344, "Target Field (T)"=w345, "Instrument.Oxford1820 in"=w346) -> ("error out"=w342:errorcluster, "Instrument.Oxford1820 out"=w341:refnum<class "Instrument.Oxford1820.lvclass">)  [unwired: 6 in]
                n118 = case shown="True" w343 {
                  tunnel: w342 -> [w352 w356]
                  tunnel: w341 -> [w351 w355]
                  tunnel: [w352 w354] -> w340
                  tunnel: [w351 w353] -> w339
                  frame False {
                  }
                  frame True {
                    n119 = call "Set Persistent Mode.vi"("error in (no error)"=w356, "Instrument.Oxford1820 in"=w355) -> ("error out"=w354:errorcluster, "Instrument.Oxford1820 out"=w353:refnum<class "Instrument.Oxford1820.lvclass">)  [unwired: 8 in]
                  }
                }
              }
              frame True {
                # "If Magnet == Target, do nothing"
              }
            }
            n120 = call <vilib>:"Add State(s) to Queue__jki_lib_state_machine.vi"("State(s) in (\"\")"=w338) -> ("States Out"=w337:string)  [unwired: 14 in]
          }
          frame "Sequence: Switch" {
            # "#todo: add abort public method"
            # "#todo: make these separate states\n1. check B = Target?\n2. Turn on switch\n3. set PSU to target\n4. check hold OR psu = target\n5. set persist mode"
            n121 = Unbundle By Name(w363) -> ("Running Step"=w365:i32, "Self Reference"=w366:refnum<class "Instrument.Oxford1820.lvclass">)
            n122 = case shown="\"Off\", Default" w361 {
              tunnel: [T5 "OFF" ("Switch Heater") T5 "ON" ("Switch Heater")] -> w360
              frame "Off", Default {
              }
              frame "On" {
              }
            }
            n123 = call "Set Switch Heater.vi"("error in (no error)"=w367, "Switch Heater"=w360, "Instrument.1820 in"=w366) -> ("error out"=w359:errorcluster)  [unwired: 6 in, 2 out]
            n124 = Increment(x=w365) -> (x+1=w364:i32)
            n125 = Bundle By Name(cluster=w363, "Running Step"=w364) -> (w362:T6)
            n126 = call <vilib>:"Add State(s) to Queue__jki_lib_state_machine.vi"("State(s) in (\"\")"=w370) -> ("States Out"=w369:string)  [unwired: 14 in]
          }
          frame "Sequence: Wait" {
            n127 = Unbundle By Name(w385) -> ("Running Step"=w383:i32)
            n128 = Equal?(x=w373, y="RESET") -> (x = y?=w374:bool)
            n129 = case shown="False" w374 {
              tunnel: [u32 10000 ("time (ms)") w391] -> w377
              tunnel: [w389 w394] -> w376
              tunnel: w375 -> [w389 w393]
              tunnel: w373 -> [_ w392]
              frame False {
              }
              frame True {
                n130 = Scan From String(format string="%d", input string=w392, error in=w393) -> (error out=w394:errorcluster, output 1=w395:i32)  [unwired: 2 in, 2 out]
                n131 = To Unsigned Long Integer(number=w395) -> (unsigned 32bit integer=w391:u32)
              }
            }
            n132 = call <userlib>:"Periodic Trigger__ogtk.vi"("time (ms)"=w377, "reset"=w374) -> ("Triggered"=w380:bool)  [unwired: 11 in, 2 out]
            n133 = Increment(x=w383) -> (x+1=w382:i32)
            n134 = Or(x=w380, y=w374) -> (x .or. y?=w379:bool)
            n135 = Select(t=w382, s=w379, f=w383) -> (s? t:f=w381:i32)
            n136 = Bundle By Name(cluster=w385, "Running Step"=w381) -> (w384:T6)
            n137 = call <vilib>:"Add State(s) to Queue__jki_lib_state_machine.vi"("State(s) in (\"\")"=w388) -> ("States Out"=w387:string)  [unwired: 14 in]
          }
          frame "Sequence: Ramp PSU to Target" {
            # "#todo: add abort public method"
            # "#todo: make these separate states\n1. check B = Target?\n2. Turn on switch\n3. set PSU to target\n4. check hold OR psu = target\n5. set persist mode"
            n138 = Unbundle By Name(w404) -> ("Running Step"=w402:i32, "Self Reference"=w397:refnum<class "Instrument.Oxford1820.lvclass">, "Field (T)"=w398:dbl, "Field Rate (T/min)"=w399:dbl)
            n139 = call "Get PSU Field.vi"("error in (no error)"=w406, "Instrument.1820 in"=w397) -> ("error out"=w405:errorcluster, "PSU Field (T)"=w408:dbl, "Instrument.1820 in"=w407:refnum<class "Instrument.Oxford1820.lvclass">)  [unwired: 7 in]
            n140 = Increment(x=w402) -> (x+1=w401:i32)
            n141 = call "Instrument.1820.FloatApprox.vi"("y"=w398, "x"=w408) -> ("x ~ y?"=w409:bool)  [unwired: 4 in]
            n142 = case shown="False" w409 {
              tunnel: [w413 w422] -> _
              tunnel: [w415 w421] -> w400
              tunnel: w407 -> [w418 w422]
              tunnel: w405 -> [w417 w421]
              tunnel: w398 -> [w420 _]
              tunnel: w399 -> [w419 _]
              frame False {
                n143 = call "Set Target.vi"("error in (no error)"=w417, "Target Rate (T/min)"=w419, "Target Field (T)"=w420, "Instrument.1820 in"=w418) -> ("error out"=w416:errorcluster, "Instrument.1820 in"=w414:refnum<class "Instrument.Oxford1820.lvclass">)  [unwired: 5 in, 1 out]
                n144 = call "Ramp to Set.vi"("error in (no error)"=w416, "Instrument.1820 in"=w414) -> ("error out"=w415:errorcluster, "Instrument.1820 in"=w413:refnum<class "Instrument.Oxford1820.lvclass">)  [unwired: 7 in, 1 out]
              }
              frame True {
                # "If PSU Field == Target, do nothing"
              }
            }
            n145 = Bundle By Name(cluster=w404, "Running Step"=w401) -> (w403:T6)
            n146 = call <vilib>:"Add State(s) to Queue__jki_lib_state_machine.vi"("State(s) in (\"\")"=w412) -> ("States Out"=w411:string)  [unwired: 14 in]
          }
          frame "Sequence: Ramp PSU to Zero" {
            # "#todo: add abort public method"
            # "#todo: make these separate states\n1. check B = Target?\n2. Turn on switch\n3. set PSU to target\n4. check hold OR psu = target\n5. set persist mode"
            n147 = Unbundle By Name(w429) -> ("Running Step"=w427:i32, "Self Reference"=w425:refnum<class "Instrument.Oxford1820.lvclass">)
            n148 = call "Ramp to Zero.vi"("error in (no error)"=w424, "Instrument.1820 in"=w425) -> ("error out"=w423:errorcluster)  [unwired: 7 in, 2 out]
            n149 = Increment(x=w427) -> (x+1=w426:i32)
            n150 = Bundle By Name(cluster=w429, "Running Step"=w426) -> (w428:T6)
            n151 = call <vilib>:"Add State(s) to Queue__jki_lib_state_machine.vi"("State(s) in (\"\")"=w432) -> ("States Out"=w431:string)  [unwired: 14 in]
          }
          frame "Sequence: Check Hold" {
            n152 = Unbundle By Name(w435) -> ("Running Step"=w437:i32, "Self Reference"=w442:refnum<class "Instrument.Oxford1820.lvclass">)
            n153 = call "Get Status.vi"("error in (no error)"=w441, "Instrument.1820 in"=w442) -> ("error out"=w440:errorcluster, "Status"=w439:T10)  [unwired: 6 in, 2 out]
            n154 = Unbundle By Name(w439) -> ("Holding"=w434:bool)
            n155 = Increment(x=w437) -> (x+1=w438:i32)
            n156 = Select(t=w438, s=w434, f=w437) -> (s? t:f=w436:i32)
            n157 = Bundle By Name(cluster=w435, "Running Step"=w436) -> (w433:T6)
            n158 = call <vilib>:"Add State(s) to Queue__jki_lib_state_machine.vi"("State(s) in (\"\")"=w445) -> ("States Out"=w444:string)  [unwired: 14 in]
          }
          frame "Sequence: Check PSU at Zero" {
            n159 = Unbundle By Name(w456) -> ("Running Step"=w448:i32, "Self Reference"=w452:refnum<class "Instrument.Oxford1820.lvclass">)
            n160 = call "Get PSU Field.vi"("error in (no error)"=w451, "Instrument.1820 in"=w452) -> ("error out"=w450:errorcluster, "PSU Field (T)"=w454:dbl)  [unwired: 7 in, 1 out]
            n161 = call "Instrument.1820.FloatApprox.vi"("y"=0.0, "x"=w454) -> ("x ~ y?"=w447:bool)  [unwired: 4 in]
            n162 = Increment(x=w448) -> (x+1=w449:i32)
            n163 = Select(t=w449, s=w447, f=w448) -> (s? t:f=w446:i32)
            n164 = Bundle By Name(cluster=w456, "Running Step"=w446) -> (w455:T6)
            n165 = call <vilib>:"Add State(s) to Queue__jki_lib_state_machine.vi"("State(s) in (\"\")"=w459) -> ("States Out"=w458:string)  [unwired: 14 in]
          }
          frame "Sequence: Set Persistent Mode" {
            # "#todo\ndelete this state"
            # "#todo: add abort public method"
            # "#todo: make these separate states\n1. check B = Target?\n2. Turn on switch\n3. set PSU to target\n4. check hold OR psu = target\n5. set persist mode"
            n166 = Unbundle By Name(w464) -> ("Self Reference"=w463:refnum<class "Instrument.Oxford1820.lvclass">, "persistent"=w460:bool)
            n167 = case shown="True" w460 {
              tunnel: w463 -> [_ w471]
              tunnel: w462 -> [w468 w470]
              tunnel: [w468 w469] -> w461
              frame False {
              }
              frame True {
                n168 = call "Set Persistent Mode.vi"("error in (no error)"=w470, "Instrument.Oxford1820 in"=w471) -> ("error out"=w469:errorcluster)  [unwired: 8 in, 1 out]
              }
            }
            n169 = call <vilib>:"Add State(s) to Queue__jki_lib_state_machine.vi"("State(s) in (\"\")"=w467) -> ("States Out"=w466:string)  [unwired: 14 in]
          }
        }
      }
    }
    frame Error {
    }
  }
  n170 = call-parent "Process.vi"("error in"=w7, "Instrument"=w6) -> ("error out"=w4:errorcluster, "Instrument out"=→"Instrument.Example out":refnum<class "Instrument.Oxford1820.lvclass">)  [unwired: 8 in]
  n171 = Merge Errors(w4, w3) -> (→"error out":errorcluster)
